vi "temp_subvi.vi"() -> ()   [LabVIEW 2019]
panel:
  in  "Length of the FCM (m)":dbl
  in  "Radius of disk (m)":dbl
  in  "Number of Disks":dbl
  in  "Tip position":dbl[](array[numeric])
  out "L1 (m)":dbl
  out "L2 (m)":dbl
  out "L3 (m)":dbl
  in  "Radius of pulley (mm)":dbl
  out "Theta 1":dbl
  out "Theta 2":dbl
  out "Theta 3":dbl
  in  "Position Reset":bool
  out "output variable":dbl
  out "output variable 2":dbl
  out "output variable 3":dbl
  out "alpha":dbl
  out "L_v":dbl
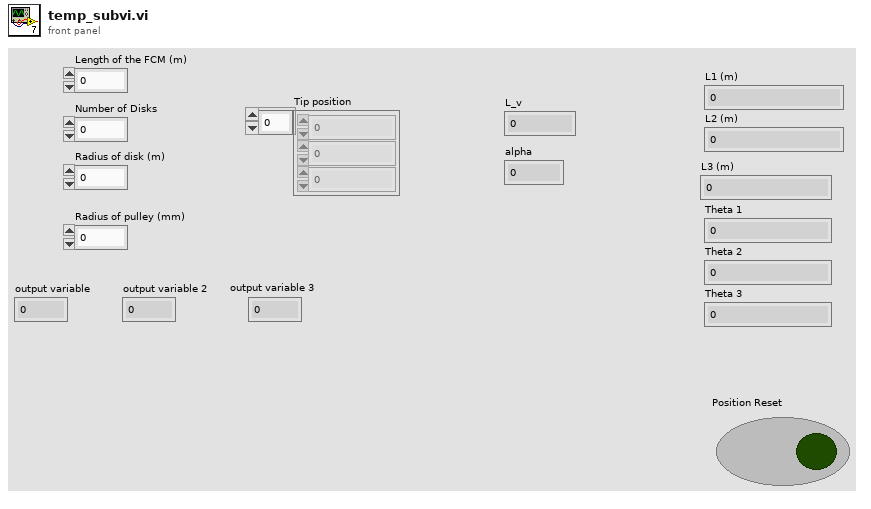
[diagram p1: front panel]
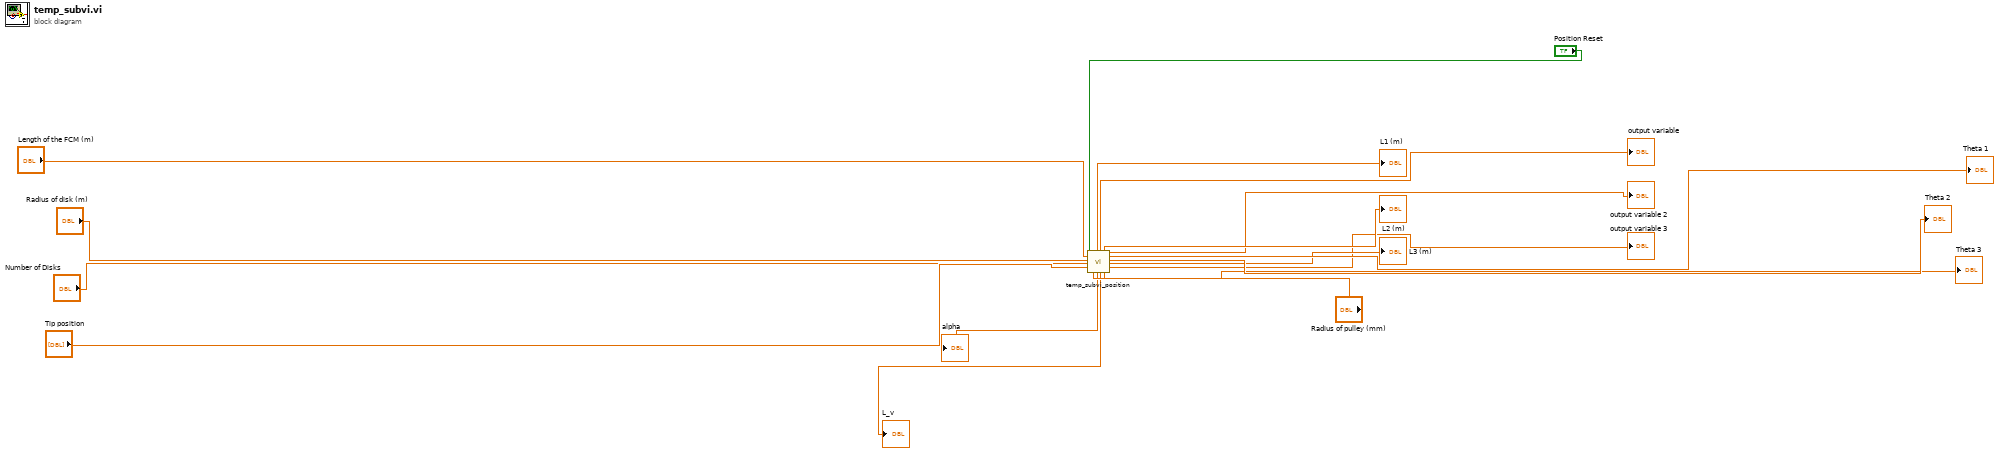
[diagram p0: block diagram]
diagram:
  n1 = call "temp_subvi_position.vi"("Position Reset"="Position Reset", "Length of the FCM (m)"="Length of the FCM (m)", "Radius of disk (m)"="Radius of disk (m)", "Number of Disks"="Number of Disks", "Tip position"="Tip position", "Radius of pulley (mm)"="Radius of pulley (mm)") -> ("L1 (m)"=→"L1 (m)":dbl, "alpha"=→"alpha":dbl, "output variable"=→"output variable":dbl, "L_v"=→"L_v":dbl, "L2 (m)"=→"L2 (m)":dbl, "Theta 3"=→"Theta 3":dbl, "output variable 2"=→"output variable 2":dbl, "Theta 1"=→"Theta 1":dbl, "Theta 2"=→"Theta 2":dbl, "L3 (m)"=→"L3 (m)":dbl, "output variable 3"=→"output variable 3":dbl)  [unwired: 3 in]
